vi "Construct Routine.vi"(8 "error in (no error)":errorcluster, 10 "Modules":refnum<class "Module.lvclass">[](array[class]), 11 "Database Assembly in":refnum<class "Database Assembly.lvclass">) -> (0 "error out":errorcluster, 3 "Database Assembly out":refnum<class "Database Assembly.lvclass">)   [LabVIEW 2020, in "Database Assembly.lvclass"]
uses:
  Database Assembly.lvclass
  C:/Users/hep/Documents/CMU gantry/Classes/Assembly/Assembly Run.lvclass
  Module/Module.lvclass
  Workspace/Fixture Enum.ctl
  Routine/Routine Enum.ctl
  Module/Module.lvclass/Module.ctl
  Database Assembly.lvclass/Database Assembly.ctl
  Module/Read Module Top Layer.vi
  Routine/Routine.lvclass
  Workspace/Fixture.lvclass
  Assembly Run.lvclass
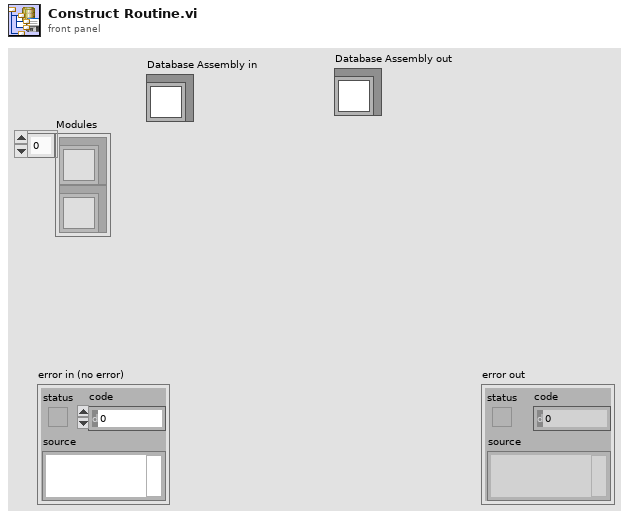
[diagram p1: front panel]
types:
  T1 = typedef "Routine.lvclass/Routine Enum.ctl" = enum16{"Primary Pick Up", "Pick Up All", "Put Down Secondary", "Put Down All", "Release Syringe", "Secondary Pick Up", "Secure Syringe", "Dispense on Plate", "Dispense on Kapton", "Dispense on Sensor"}
  T2 = typedef "Fixture.lvclass/Fixture Enum.ctl" = enum16{"Assembly Tray", "Syringe Space", "Component", "Pick Up Tool", "Current Position"}
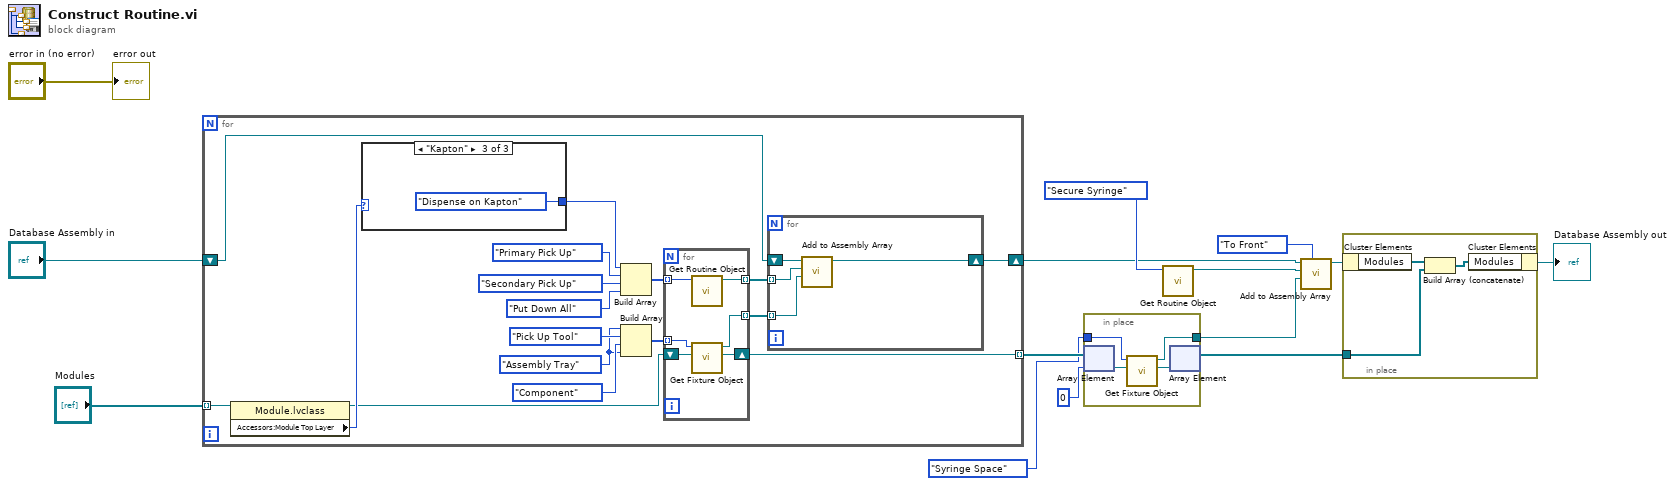
[diagram p0: block diagram]
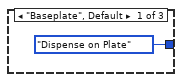
[diagram p2: hidden frame]
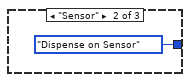
[diagram p3: hidden frame]
diagram:
  n1 = for {
    tunnel: "Modules" -> [w31] mode=indexing
    tunnel: [w15] -> w6 mode=indexing
    shift-right: [w20] -> w9
    shift-left: "Database Assembly in" -> [w19]
    w25 = Fixture_Enum."Assembly Tray" ("Fixture")
    n2 = property class="Module.lvclass"(reference=w31) -> (reference out=w16:refnum<class "Module.lvclass">, "Accessors:Module Top Layer"=w21:enum16{"Baseplate", "Kapton", "Sensor", "PCB"})  [unwired: 1 in, 1 out]
    n3 = case shown="\"Kapton\"" w21 {
      tunnel: [Routine_Enum."Dispense on Plate" ("Routine") Routine_Enum."Dispense on Sensor" ("Routine") Routine_Enum."Dispense on Kapton" ("Routine")] -> w22
      frame "Baseplate", Default {
      }
      frame "Sensor" {
      }
      frame "Kapton" {
      }
    }
    n4 = Build Array(w22, Routine_Enum."Primary Pick Up" ("Routine"), Routine_Enum."Secondary Pick Up" ("Routine"), Routine_Enum."Put Down All" ("Routine")) -> (w24:T1[])
    n5 = Build Array(w25, Fixture_Enum."Pick Up Tool" ("Fixture"), Fixture_Enum."Component" ("Fixture"), w25) -> (w23:T2[])
    n6 = for {
      tunnel: w24 -> [w40] mode=indexing
      tunnel: [w38] -> w17 mode=indexing
      tunnel: w23 -> [w39] mode=indexing
      tunnel: [w37] -> w18 mode=indexing
      shift-right: [w35] -> w15
      shift-left: w16 -> [w36]
      n7 = call "Get Routine Object.vi"("Routine"=w40) -> ("Routine out"=w38:refnum<class "Routine.lvclass">)  [unwired: 9 in, 1 out]
      n8 = call "Get Fixture Object.vi"("Module In"=w36, "Fixture"=w39) -> ("Module Out"=w35:refnum<class "Module.lvclass">, "Workspace.lvclass"=w37:refnum<class "Fixture.lvclass">)  [unwired: 7 in, 1 out]
    }
    n9 = for {
      tunnel: w17 -> [w44] mode=indexing
      tunnel: w18 -> [w43] mode=indexing
      shift-right: [w41] -> w20
      shift-left: w19 -> [w42]
      n10 = call "Add to Assembly Array.vi"("Workspace In"=w43, "Routine In"=w44, "Assembly Run in"=w42) -> ("Assembly Run out"=w41:refnum<class "Database Assembly.lvclass">)  [unwired: 7 in, 1 out]
    }
  }
  n11 = in-place {
    in-place-border: Fixture_Enum."Syringe Space" ("Fixture") -> [w48]
    in-place-border: [w45] -> w4
    n12 = in-place-array #1(w6, 0) -> (w47:refnum<class "Module.lvclass">)
    n13 = call "Get Fixture Object.vi"("Module In"=w47, "Fixture"=w48) -> ("Module Out"=w46:refnum<class "Module.lvclass">, "Workspace.lvclass"=w45:refnum<class "Fixture.lvclass">)  [unwired: 7 in, 1 out]
    n14 = in-place-array #1(w46) -> (w3:refnum<class "Module.lvclass">[])  [unwired: 1 out]
  }
  n15 = call "Get Routine Object.vi"("Routine"=Routine_Enum."Secure Syringe") -> ("Routine out"=w11:refnum<class "Routine.lvclass">)  [unwired: 9 in, 1 out]
  n16 = call "Add to Assembly Array.vi"("Type"=enum16{"To End", "To Front"}."To Front", "Workspace In"=w4, "Routine In"=w11, "Assembly Run in"=w9) -> ("Assembly Run out"=w8:refnum<class "Database Assembly.lvclass">)  [unwired: 6 in, 1 out]
  n17 = in-place {
    in-place-border: w3 -> [w50]
    n18 = in-place-cluster #2(w8) -> ("Modules"=w51:refnum<class "Module.lvclass">[])
    n19 = Build Array (concatenate)(w51, w50) -> (w49:refnum<class "Module.lvclass">[])
    n20 = in-place-cluster #2("Modules"=w49) -> (→"Database Assembly out":refnum<class "Database Assembly.lvclass">)
  }
  "error out" <- "error in (no error)"
